vi "SwissSPAD Live_Gate Image Data Q.vi"(1 "create if not found? (T)":bool, 4 "error in (no error)":errorcluster, 6 "SwissSPAD Live Gate Image Data Q Name":string="SS2 Live Gate Data Q") -> (3 "created new Gate Image Data Q?":bool, 5 "error out":errorcluster, 7 "SwissSPAD Live Gate Image Data Q":refnum<queue>)   [LabVIEW 2021]
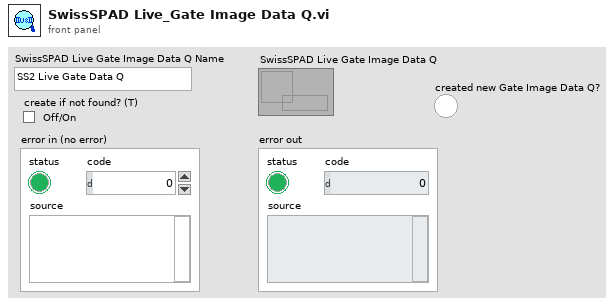
[diagram p1: front panel]
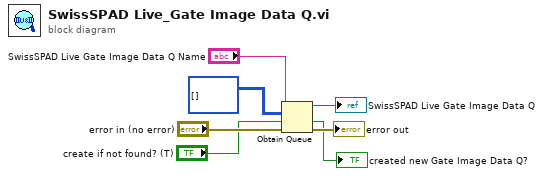
[diagram p0: block diagram]
diagram:
  n1 = Obtain Queue(name (unnamed)="SwissSPAD Live Gate Image Data Q Name", element data type=u8[][] [] ("second subarray"), create if not found? (T)="create if not found? (T)", error in (no error)="error in (no error)") -> (queue out=→"SwissSPAD Live Gate Image Data Q":refnum<queue>, created new?=→"created new Gate Image Data Q?":bool, error out=→"error out":errorcluster)  [unwired: 1 in]
